vi "read_rn16_v2.vi"() -> ()   [LabVIEW 2015]
panel:
  out "0, 1":i16[](array[numeric])
  out "RN16 Chart":i16(graph)
  in  "threshold":dbl=0.004
  in  "low":dbl=0.175
  in  "high":dbl=0.215
  out "RN16 Graph":dynamicdata(graph)
  in  "x factor":dbl=0.2
  in  "avg factor":dbl=0.8
  out "Around RN16":dynamicdata(graph) caption="Signals"
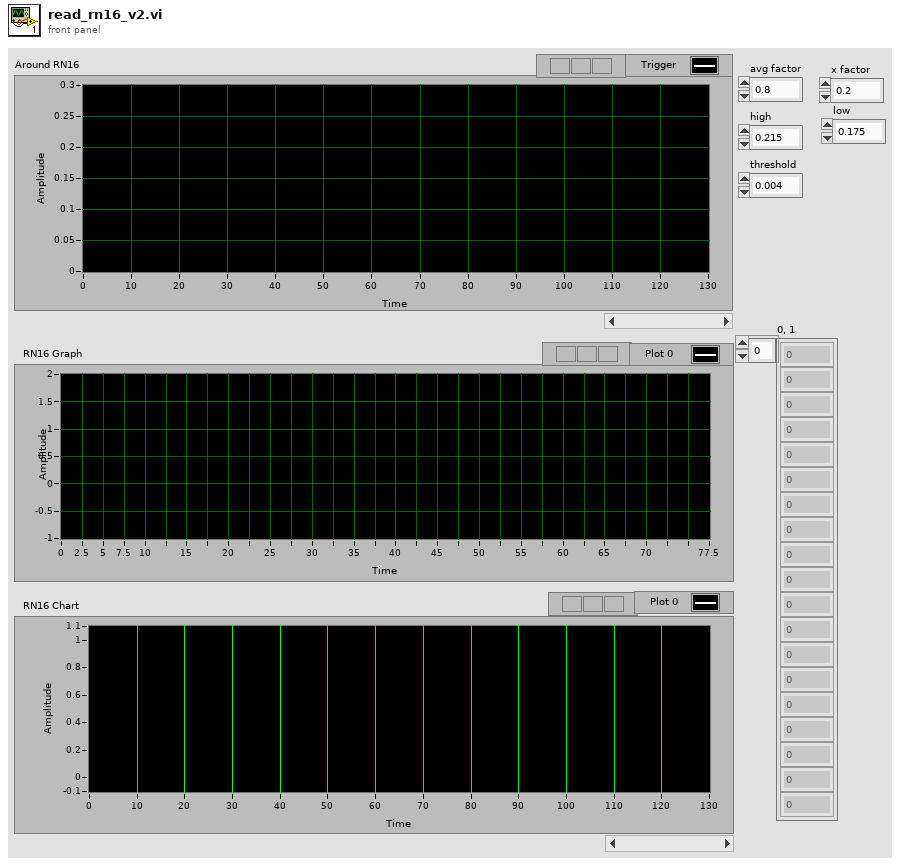
[diagram p1: front panel]
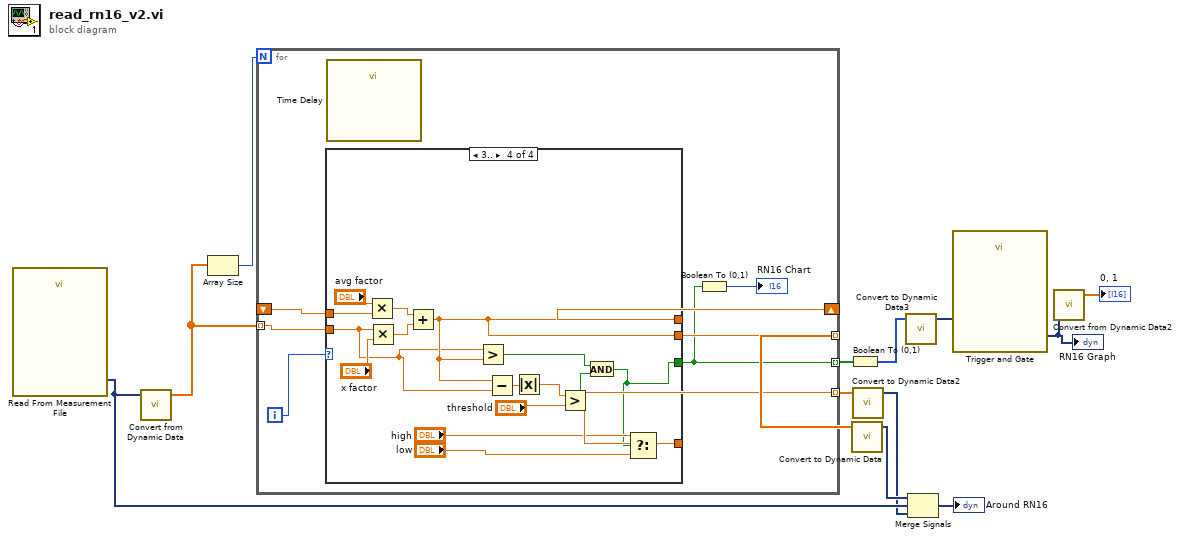
[diagram p0: block diagram]
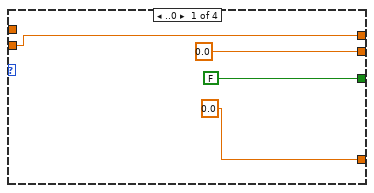
[diagram p2: hidden frame]
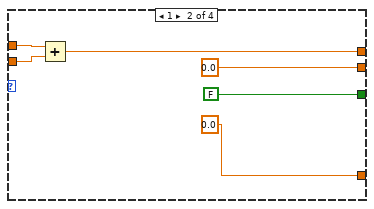
[diagram p3: hidden frame]
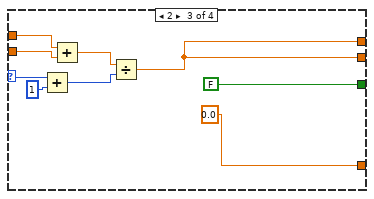
[diagram p4: hidden frame]
diagram:
  n1 = call "Read From Measurement File"() -> ("Signals"=w10:dynamicdata)  [unwired: 6 in, 5 out]
  n2 = call "Convert from Dynamic Data"("Dynamic Data Type"=w10) -> ("Array"=w12:dbl[])  [unwired: 3 in]
  n3 = Array Size(array=w12) -> (size(s)=w13:i32)
  n4 = for {
    N: w13 -> [_]
    tunnel: w12 -> [w15] mode=indexing
    tunnel: [w20] -> w11 mode=indexing
    shift-right: [w18] -> _
    shift-left: _ -> [w19]
    tunnel: [w16] -> w7 mode=indexing
    tunnel: [w17] -> w6 mode=indexing
    i -> [w21]
    n5 = case shown="3.." w21 {
      selector: w21 -> [_ _ w37 _]
      tunnel: w15 -> [w24 w30 w36 w44]
      tunnel: [0.0 0.0 w34 w45] -> w20
      tunnel: w19 -> [_ w31 w35 w56]
      tunnel: [w24 w28 w34 w45] -> w18
      tunnel: [FALSE FALSE FALSE w41] -> w16
      tunnel: [0.0 ("low") 0.0 ("low") 0.0 ("low") w50] -> w17
      frame ..0 {
      }
      frame 1 {
        n6 = Add(x=w31, y=w30) -> (x+y=w28:dbl)
      }
      frame 2 {
        n7 = Add(x=w37, y=1) -> (x+y=w38:i32)
        n8 = Add(x=w35, y=w36) -> (x+y=w39:dbl)
        n9 = Divide(x=w39, y=w38) -> (x/y=w34:dbl)
      }
      frame 3.. {
        n10 = Multiply(x="avg factor", y=w56) -> (x*y=w53:dbl)
        n11 = Multiply(x=w44, y="x factor") -> (x*y=w52:dbl)
        n12 = Add(x=w53, y=w52) -> (x+y=w45:dbl)
        n13 = Greater?(x=w44, y=w45) -> (0:w42:bool)
        n14 = Subtract(x=w45, y=w44) -> (x-y=w48:dbl)
        n15 = Absolute Value(x=w48) -> (abs(x)=w47:dbl)
        n16 = Greater?(x=w47, y="threshold") -> (0:w43:bool)
        n17 = And(x=w42, y=w43) -> (x .and. y?=w41:bool)
        n18 = Select(t="high", s=w41, f="low") -> (s? t:f=w50:dbl)
      }
    }
    n19 = call "Time Delay"() -> ()  [unwired: 11 in, 1 out]
    n20 = Boolean To (0,1)(Boolean=w16) -> (0, 1=→"RN16 Chart":i16)
  }
  n21 = Boolean To (0,1)(Boolean=w7) -> (0, 1=w4:i16[])
  n22 = call "Convert to Dynamic Data"("Array"=w11) -> ("Dynamic Data Type"=w8:dynamicdata)  [unwired: 3 in]
  n23 = call "Convert to Dynamic Data2"("Array"=w6) -> ("Dynamic Data Type"=w5:dynamicdata)  [unwired: 3 in]
  n24 = call "Convert to Dynamic Data3"("Array"=w4) -> ("Dynamic Data Type"=w3:dynamicdata)  [unwired: 3 in]
  n25 = Merge Signals(w8, w10, w5) -> (→"Around RN16":dynamicdata)
  n26 = call "Trigger and Gate"("Signals"=w3) -> ("Triggered Signals"=w2:dynamicdata)  [unwired: 7 in, 3 out]
  "RN16 Graph" <- w2
  n27 = call "Convert from Dynamic Data2"("Dynamic Data Type"=w2) -> ("Array"=→"0, 1":dbl[])  [unwired: 3 in]
